vi "Init.vi"(8 "Project:Active Project":refnum<vi>, 9 "Application Instance":refnum<vi>, 10 "Name":string, 11 "Second Library Script Strategy in":refnum<class "Second Library Script Strategy.lvclass">) -> (3 "Second Library Script Strategy out":refnum<class "Second Library Script Strategy.lvclass">)   [LabVIEW 2021, in "_Create From Template.lvlib" / "Script Strategy.lvlib" / "Second Library Script Strategy.lvclass"]
uses:
  Second Library Script Strategy.lvclass
  Second Library Script Strategy.lvclass/Second Library Script Strategy.ctl
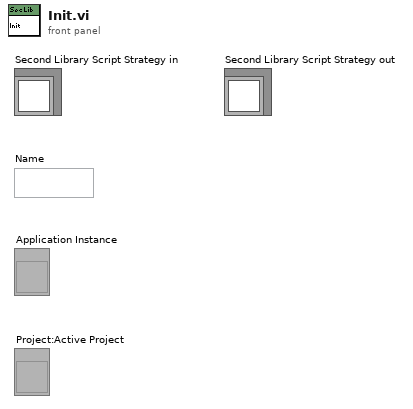
[diagram p1: front panel]
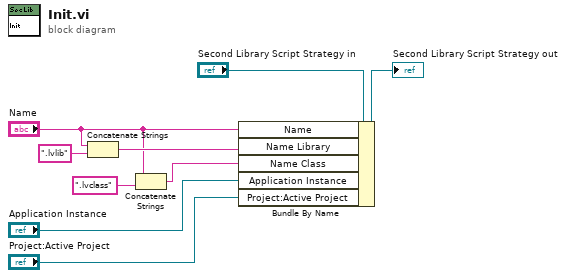
[diagram p0: block diagram]
diagram:
  n1 = Concatenate Strings("Name", ".lvlib" ("string")) -> (w7:string)
  n2 = Concatenate Strings("Name", ".lvclass" ("regular expression")) -> (w5:string)
  n3 = Bundle By Name(cluster="Second Library Script Strategy in", "Name"="Name", "Name Library"=w7, "Name Class"=w5, "Application Instance"="Application Instance", "Project:Active Project"="Project:Active Project") -> (→"Second Library Script Strategy out":refnum<class "Second Library Script Strategy.lvclass">)
